vi "SaveParams.vi"(0 "Variables":T1={"Number of rings"=1, "sound spd (cm/s)"=150000, "z span (cm)"=4.0, "z steps"=20, "y spacing (cm)"=0.01, "y steps"=50, "time step (s)"=1e-08, "z"=0.0, "y"=0.0, "ref delay"=0.0, "freq (MHz)"=4.71, "cycles"=300} {"freq (MHz)" format="%.2f"; "z span (cm)" format="%.2f"; "y" format="%.2f"; "ref delay" format="%.2f"; "y spacing (cm)" format="%.3f"; "z" format="%.2f"; "time step (s)" format="%.2e"}, 1 "Trans Geometry":T2={"Radius (cm)"=12.0, "a (cm)"=2.5, "focus location"=12.0} {"focus location" format="%.2f"; "a (cm)" format="%.2f"; "Radius (cm)" format="%.2f"}, 2 "Path":path) -> ()   [LabVIEW 2022 SP3]
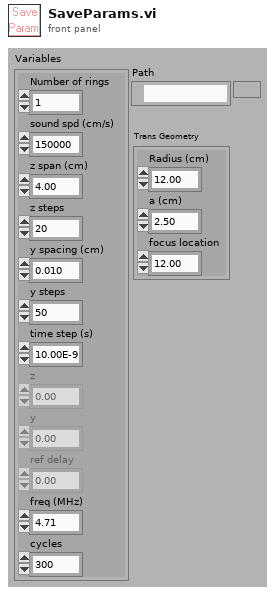
[diagram p1: front panel]
types:
  T1 = cluster{"Number of rings":i32, "sound spd (cm/s)":i32, "z span (cm)":dbl, "z steps":i32, "y spacing (cm)":dbl, "y steps":i32, "time step (s)":sgl, "z":dbl, "y":dbl, "ref delay":dbl, "freq (MHz)":dbl, "cycles":i32}
  T2 = cluster{"Radius (cm)":dbl, "a (cm)":dbl, "focus location":dbl}
  T3 = cluster{"Number of rings":dbl, "sound spd (cm/s)":dbl, "z span (cm)":dbl, "z steps":dbl, "y spacing (cm)":dbl, "y steps":dbl, "time step (s)":dbl, "z":dbl, "y":dbl, "ref delay":dbl, "freq (MHz)":dbl, "cycles":dbl}
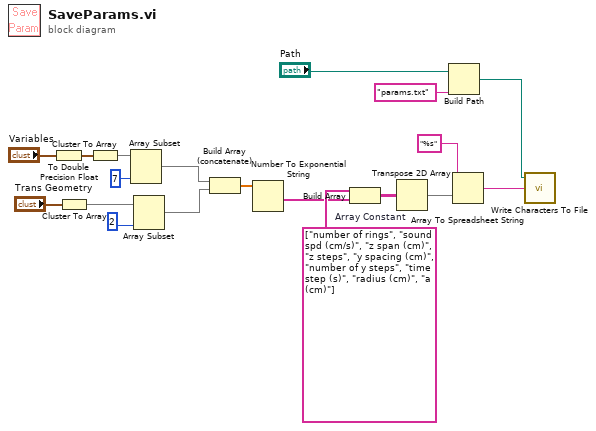
[diagram p0: block diagram]
diagram:
  w12 = string[] ["number of rings", "sound spd (cm/s)", "z span (cm)", "z steps", "y spacing (cm)", "number of y steps", "time step (s)", "radius (cm)", "a (cm)"]  # Array Constant
  n1 = To Double Precision Float(number="Variables") -> (double precision float=w2:T3)
  n2 = Cluster To Array(cluster="Trans Geometry") -> (array=w7:dbl[])
  n3 = Cluster To Array(cluster=w2) -> (array=w3:dbl[])
  n4 = Array Subset(array=w3, length=7) -> (w8:dbl[])  [unwired: 1 in]
  n5 = Array Subset(array=w7, length=2) -> (w9:dbl[])  [unwired: 1 in]
  n6 = Build Array (concatenate)(w8, w9) -> (w10:dbl[])
  n7 = Number To Exponential String(number=w10) -> (E-format string=w11:string[])  [unwired: 3 out]
  n8 = Build Array(w12, w11) -> (w13:string[][])
  n9 = Transpose 2D Array(2D array=w13) -> (transposed array=w14:string[][])
  n10 = Build Path(base path="Path", name or relative path="params.txt") -> (appended path=w19:path)
  n11 = Array To Spreadsheet String(array=w14, 3:"%s") -> (spreadsheet string=w16:string)  [unwired: 1 out]
  n12 = call <vilib>:"Write Characters To File.vi"("character string"=w16, "file path (dialog if empty)"=w19) -> ()  [unwired: 1 in, 3 out]
